vi "playsound.vi"() -> ()   [LabVIEW 2012]
panel:
  in  "Stop Button":bool
  in  "Play?":cluster{" Sound 1":bool, " Sound 2":bool}
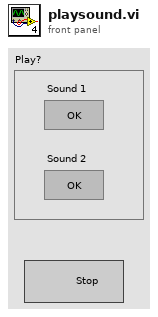
[diagram p1: front panel]
types:
  T1 = typedef "Sound Output Task ID.ctl" = u32
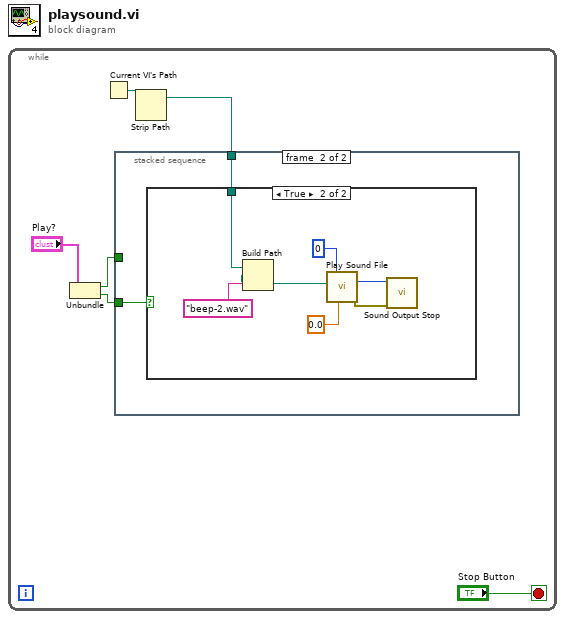
[diagram p0: block diagram]
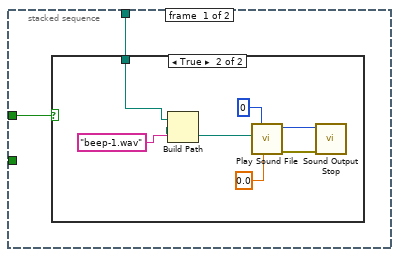
[diagram p2: hidden frame]
diagram:
  n1 = while {
    stop <- "Stop Button" stop-if-true
    n2 = Unbundle("Play?") -> ("Sound 1"=w3:bool, "Sound 2"=w2:bool)
    n3 = Current VI's Path() -> (path=w6:path)
    n4 = Strip Path(path=w6) -> (stripped path=w5:path)  [unwired: 1 out]
    n5 = stacked-sequence {
      tunnel: w5 -> [w8 w17]
      tunnel: w3 -> [w7 _]
      tunnel: w2 -> [_ w16]
      frame #0 {
        n6 = case shown="True" w7 {
          tunnel: w8 -> [_ w9]
          frame False {
          }
          frame True {
            n7 = Build Path(base path=w9, name or relative path="beep-1.wav") -> (appended path=w14:path)
            n8 = call <vilib>:"Play Sound File.vi"("timeout (sec)"=0.0, "path"=w14, "device ID"=u32 0) -> ("error out"=w10:errorcluster, "task ID"=w11:T1)  [unwired: 7 in]
            n9 = call <vilib>:"Sound Output Stop.vi"("error in (no error)"=w10, "task ID"=w11) -> ()  [unwired: 8 in, 2 out]
          }
        }
      }
      frame #1 {
        n10 = case shown="True" w16 {
          tunnel: w17 -> [_ w20]
          frame False {
          }
          frame True {
            n11 = Build Path(base path=w20, name or relative path="beep-2.wav") -> (appended path=w23:path)
            n12 = call <vilib>:"Play Sound File.vi"("timeout (sec)"=0.0, "path"=w23, "device ID"=u32 0) -> ("error out"=w18:errorcluster, "task ID"=w19:T1)  [unwired: 7 in]
            n13 = call <vilib>:"Sound Output Stop.vi"("error in (no error)"=w18, "task ID"=w19) -> ()  [unwired: 8 in, 2 out]
          }
        }
      }
    }
  }
